vi "VarGlobUIStopLoops.vi"() -> ()   [LabVIEW 2017]
panel:
  in  "StopUILoops":bool
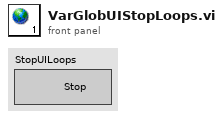
[diagram p1: front panel]
diagram:
